vi "save_system_reference_meas_hdf.vi"(7 "Device Name":tag="DAQ2", 8 "HDF path":path, 9 "TxRxParams":T1={"sample rate"=1000000.0, "Transmit frequency"=25000.0, "Transmit amplitude"=1.577, "sample rate digital out"=40000.0, "TX cycles"=600, "sample rate DAQ1"=1000000.0, "Receive frequency"=75000.0, "Receive range"=1.0, "TX harmonics"=[50000.0, 75000.0, 100000.0, 125000.0, 150000.0, 175000.0, 200000.0, 225000.0]} {"TX harmonics" format="%#_6p"; "Receive frequency" format="%#_6p"; "sample rate DAQ1" format="%#_6p"; "sample rate digital out" format="%#_6p"; "Transmit frequency" format="%#_6p"; "sample rate" format="%#_6p"}, 11 "queue out 2":refnum<queue>) -> ()   [LabVIEW 2021]
uses:
  <vilib>/UPVI/lvhdf5/file.llb/LVH5F Operation.ctl
  <vilib>/Utility/miscctls.llb/LVRectTypeDef.ctl
  <vilib>/UPVI/lvhdf5/group.llb/H5G_obj_t.ctl
  <vilib>/UPVI/lvhdf5/dataset.llb/LVH5D Operation.ctl
  <vilib>/UPVI/lvhdf5/attribute.llb/Write Multiple Attributes.vi
  <vilib>/UPVI/lvhdf5/utility.llb/Select HDF5 Dialog.vi
  <vilib>/UPVI/lvhdf5/utility.llb/Select HDF5 Dialog (Object Only).vi
  <vilib>/UPVI/lvhdf5/dataset.llb/Simple H5Dwrite (Variant).vi
  <vilib>/UPVI/lvhdf5/attribute.llb/LVH5A Operation.ctl
  <vilib>/UPVI/lvhdf5/attribute.llb/LVH5 Write Attributes.xnode
  <vilib>/UPVI/lvhdf5/library.llb/HDF5 Ref.ctl
  <vilib>/UPVI/lvhdf5/dataset.llb/Simple H5Dwrite.xnode
  <resource>/objmgr/daqmx.rc
  <vilib>/UPVI/lvhdf5/attribute.llb/Cluster to Attribute Array.xnode
  <vilib>/UPVI/lvhdf5/identifier.llb/Not an HDF5 Refnum Constant.vi
  <vilib>/Utility/error.llb/Error Cluster From Error Code.vi
  <vilib>/UPVI/lvhdf5/dataset.llb/OpenCreateReplace Dataset by Element Type.vi
  <vilib>/UPVI/lvhdf5/dataspace.llb/H5Sselect_hyperslab.vi
  <vilib>/UPVI/lvhdf5/dataset.llb/H5Dwrite (Variant).vi
  <vilib>/UPVI/lvhdf5/dataset.llb/H5Dget_space.vi
  <vilib>/UPVI/lvhdf5/attribute.llb/private/LVH5AwriteWDTAttrs.vi
  <vilib>/UPVI/lvhdf5/dataspace.llb/H5Sclose.vi
  <vilib>/UPVI/lvhdf5/dataset.llb/H5Dclose.vi
  <vilib>/UPVI/lvhdf5/utility.llb/Select HDF5 Dialog (File and Object).vi
  <vilib>/UPVI/lvhdf5/library.llb/HDF5 Ref.lvclass
  <vilib>/Utility/Data Type/Get Type Information.vi
  <vilib>/Utility/Data Type/NI_Data Type.lvlib
  <vilib>/Utility/Data Type/Get Cluster Information.vi
panel:
  out "Run description":string
  out "index":i32
  out "f_harmonics":dbl[](array[numeric])
  out "x != 0?":bool
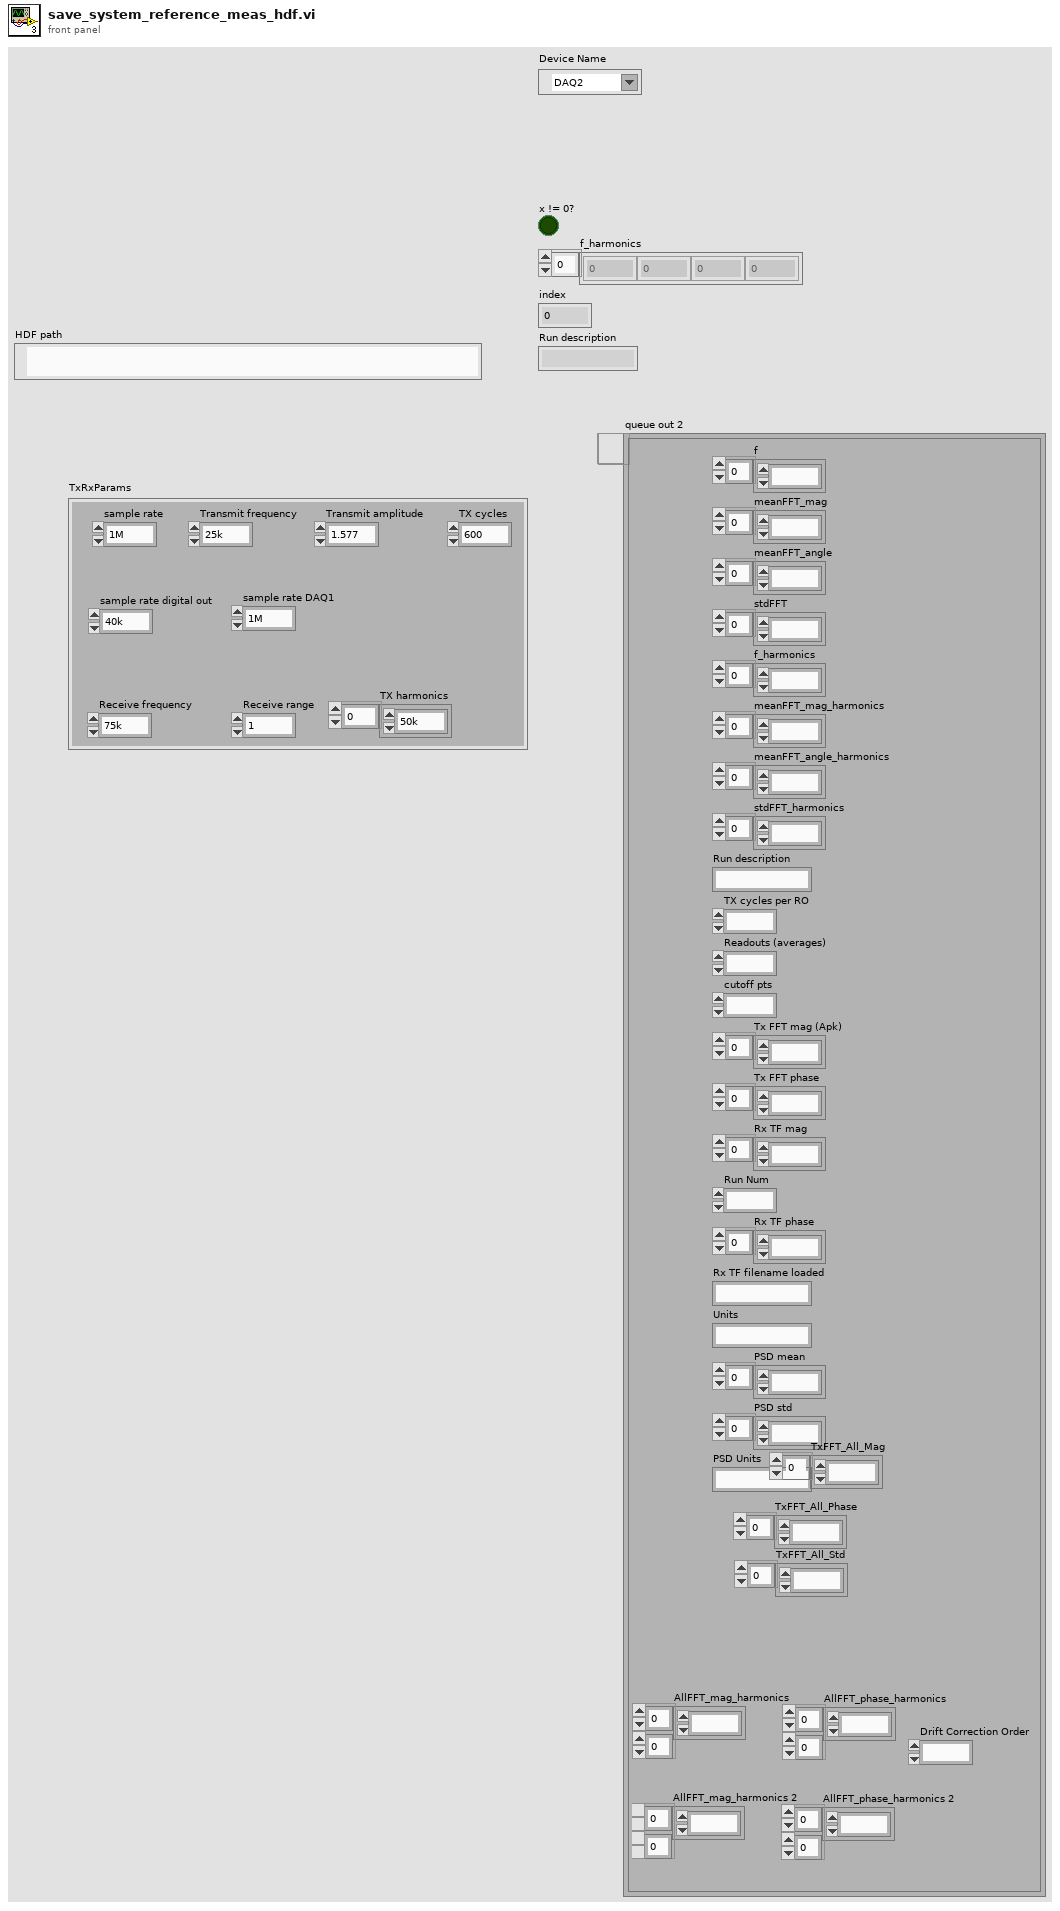
[diagram p1: front panel]
types:
  T1 = cluster{"sample rate":dbl, "Transmit frequency":dbl, "Transmit amplitude":dbl, "sample rate digital out":dbl, "TX cycles":i32, "sample rate DAQ1":dbl, "Receive frequency":dbl, "Receive range":dbl, "TX harmonics":dbl[]}
  T2 = typedef "LVH5F Operation.ctl" = enum16{"open", "open or create", "create or replace", "create or replace (with confirmation)", "create", "open (read only)"}
  T3 = typedef "LVRectTypeDef.ctl" = cluster{"Left":i16, "Top":i16, "Right":i16, "Bottom":i16}
  T4 = cluster{"Behavior":enum32{"Invalid", "Default", "Floating", "Floating/Auto-Hide", "Modal"}, "Position":T3, "Center":bool, "Title":string}
  T5 = typedef "LVH5D Operation.ctl" = enum16{"open", "replace", "create", "open or create", "create or replace", "create or replace with confirmation"}
  T6 = typedef "H5G_obj_t.ctl" = i32
  T7 = cluster{"Object Types (any)":T6[], "Object Pattern":string}
  T8 = cluster{"f":dbl[], "meanFFT_mag":dbl[], "meanFFT_angle":dbl[], "stdFFT":dbl[], "f_harmonics":dbl[], "meanFFT_mag_harmonics":dbl[], "meanFFT_angle_harmonics":dbl[], "stdFFT_harmonics":dbl[], "Run description":string, "TX cycles per RO":dbl, "Readouts (averages)":dbl, "cutoff pts":dbl, "Tx FFT mag (Apk)":dbl[], "Tx FFT phase":dbl[], "Rx TF mag":dbl[], "Run Num":i32, "Rx TF phase":dbl[], "Rx TF filename loaded":string, "Units":string, "PSD mean":dbl[], "PSD std":dbl[], "PSD Units":string, "TxFFT_All_Mag":dbl[], "TxFFT_All_Phase":dbl[], "TxFFT_All_Std":dbl[], "AllFFT_mag_harmonics":dbl[][], "AllFFT_phase_harmonics":dbl[][], "Drift Correction Order":dbl, "AllFFT_mag_harmonics 2":dbl[][], "AllFFT_phase_harmonics 2":dbl[][]}
  T9 = typedef "HDF5 Ref.ctl" = refnum<class "HDF5 Ref.lvclass">
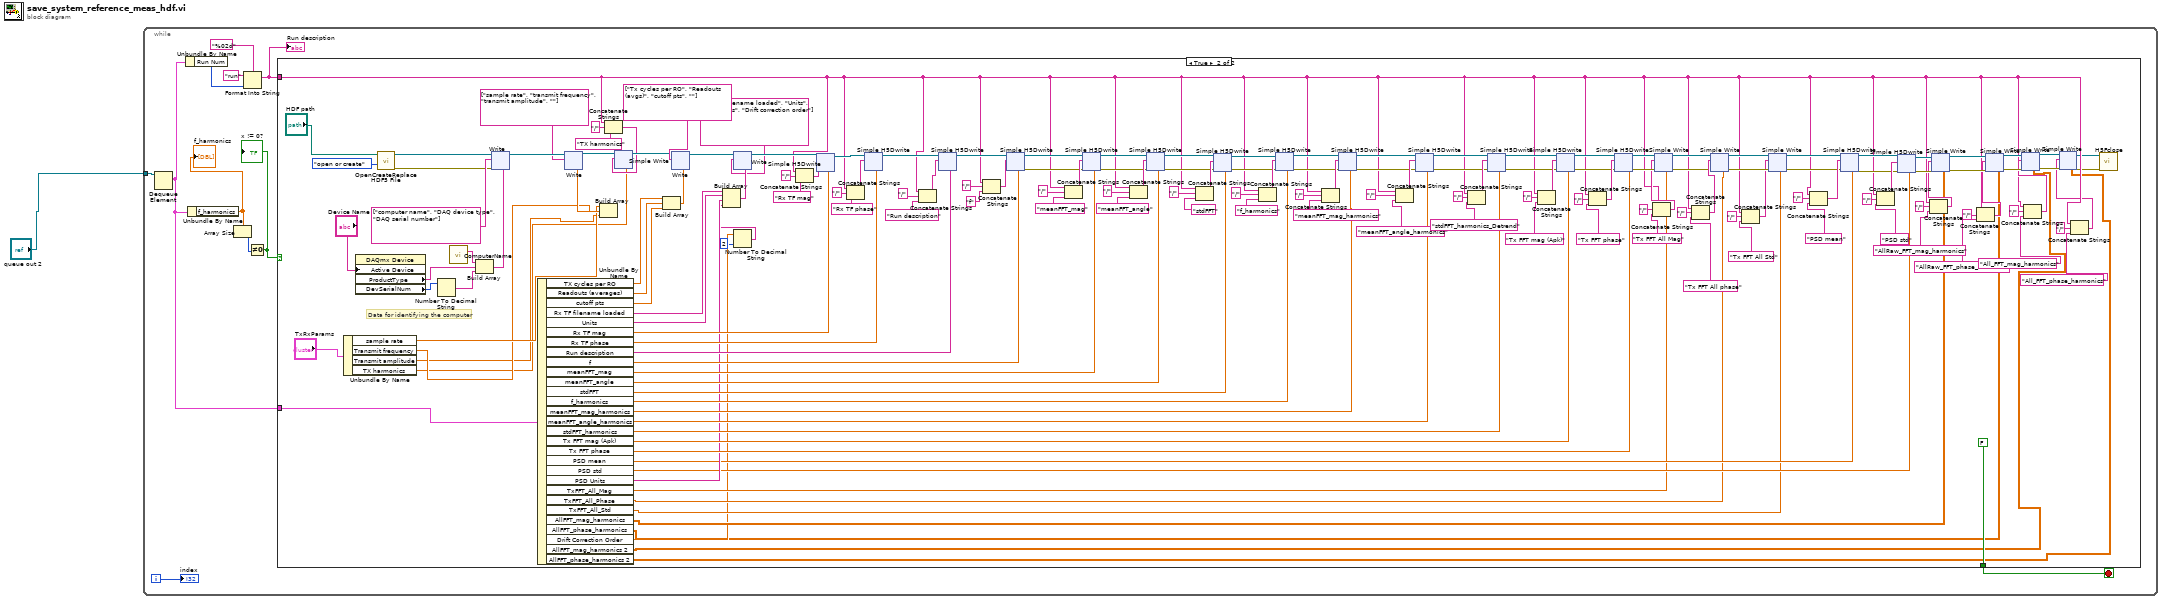
[diagram p0: block diagram]
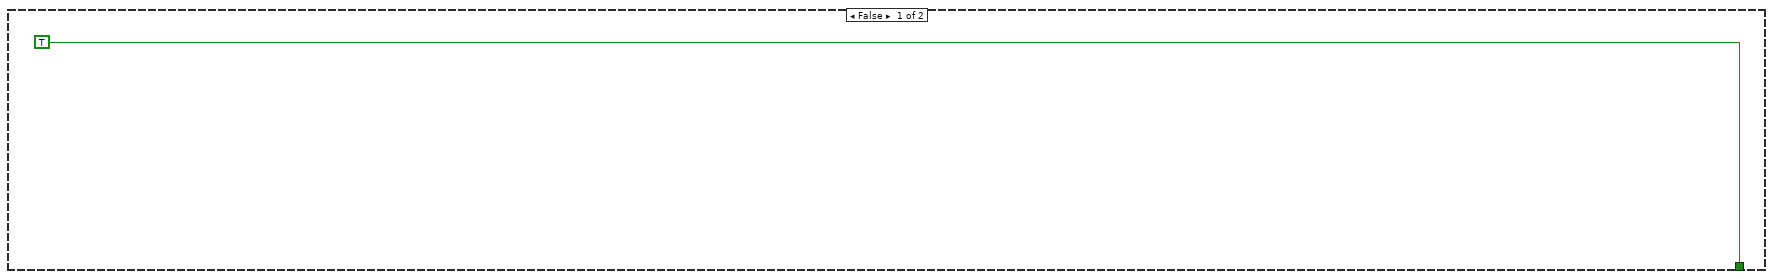
[diagram p2: hidden frame]
diagram:
  n1 = while {
    tunnel: "queue out 2" -> [w12]
    i -> [w8]
    stop <- w9 stop-if-true
    n2 = Dequeue Element(queue=w12) -> (element=w6:T8)  [unwired: 2 in, 3 out]
    n3 = Unbundle By Name(w6) -> ("Run Num"=w5:i32)
    n4 = Unbundle By Name(w6) -> ("f_harmonics"=w7:dbl[])
    "f_harmonics" <- w7
    n5 = Array Size(array=w7) -> (size(s)=w11:i32)
    n6 = Format Into String(format string="%02d", initial string="run", w5) -> (resulting string=w2:string)  [unwired: 1 in, 1 out]
    "Run description" <- w2
    n7 = Not Equal To 0?(x=w11) -> (x != 0?=w10:bool)
    "x != 0?" <- w10
    n8 = case shown="True" w10 {
      tunnel: w6 -> [_ w170]
      tunnel: [TRUE FALSE] -> w9
      tunnel: w2 -> [_ w19]
      frame False {
      }
      frame True {
        # "Data for identifying the computer"
        n9 = Unbundle By Name("TxRxParams") -> ("sample rate"=w70:dbl, "Transmit frequency"=w69:dbl, "Transmit amplitude"=w68:dbl, "TX harmonics"=w67:dbl[])
        n10 = property class="DAQmx Device"("Active Device"="Device Name") -> ("ProductType"=w181:string, "DevSerialNum"=w183:u32)  [unwired: 2 in, 2 out]
        n11 = call <vilib>:"OpenCreateReplace HDF5 File.vi"("function (open or create)"=LVH5F_Operation."open or create", "path"="HDF path") -> ("error out"=w175:errorcluster, "HDF5 Ref out"=w178:T9)  [unwired: 6 in]
        n12 = Number To Decimal String(number=w183) -> (decimal integer string=w182:string)  [unwired: 1 in]
        n13 = call "ComputerName.vi"() -> ("String/Binary data"=w180:string)  [unwired: 4 in, 1 out]
        n14 = Build Array(w180, w181, w182) -> (w177:string[])
        n15 = xnode "Write"("HDF5 Ref"=w178, "error in (no error)"=w175, "Name(s)"=string[] ["computer name", "DAQ device type", "DAQ serial number"], "Value(s)"=w177) -> ("HDF5 Ref out"=w126:T9)  [unwired: 1 in, 1 out]
        n16 = Unbundle By Name(w170) -> ("TX cycles per RO"=w112:dbl, "Readouts (averages)"=w111:dbl, "cutoff pts"=w110:dbl, "Rx TF filename loaded"=w88:string, "Units"=w90:string, "Rx TF mag"=w97:dbl[], "Rx TF phase"=w96:dbl[], "Run description"=w107:string, "f"=w140:dbl[], "meanFFT_mag"=w159:dbl[], "meanFFT_angle"=w158:dbl[], "stdFFT"=w157:dbl[], "f_harmonics"=w156:dbl[], "meanFFT_mag_harmonics"=w144:dbl[], "meanFFT_angle_harmonics"=w138:dbl[], "stdFFT_harmonics"=w137:dbl[], "Tx FFT mag (Apk)"=w120:dbl[], "Tx FFT phase"=w118:dbl[], "PSD mean"=w80:dbl[], "PSD std"=w79:dbl[], "PSD Units"=w81:string, "TxFFT_All_Mag"=w48:dbl[], "TxFFT_All_Phase"=w47:dbl[], "TxFFT_All_Std"=w46:dbl[], "AllFFT_mag_harmonics"=w33:dbl[][], "AllFFT_phase_harmonics"=w20:dbl[][], "Drift Correction Order"=w32:dbl, "AllFFT_mag_harmonics 2"=w15:dbl[][], "AllFFT_phase_harmonics 2"=w14:dbl[][])
        n17 = Build Array(w70, w69, w68) -> (w124:dbl[])
        n18 = xnode "Write"("HDF5 Ref"=w126, "Name(s)"=string[] ["sample rate", "transmit frequency", "transmit amplitude", ""], "Value(s)"=w124) -> ("HDF5 Ref out"=w86:T9)  [unwired: 2 in, 1 out]
        n19 = Concatenate Strings(w19, "/" ("string"), "TX harmonics" ("string")) -> (w82:string)
        n20 = xnode "Simple Write"("Dataset Path"=w82, "HDF5 Path or Ref"=w86, "Data"=w67) -> ("HDF5 Ref out"=w85:T9)  [unwired: 5 in, 2 out]
        n21 = Build Array(w112, w111, w110) -> (w109:dbl[])
        n22 = xnode "Write"("HDF5 Ref"=w85, "Name(s)"=string[] ["Tx cycles per RO", "Readouts (avgs)", "cutoff pts", ""], "Value(s)"=w109) -> ("HDF5 Ref out"=w92:T9)  [unwired: 2 in, 1 out]
        n23 = Number To Decimal String(number=w32, width (-)=i16 2) -> (decimal integer string=w30:string)
        n24 = Build Array(w88, w90, w81, w30) -> (w89:string[])
        n25 = xnode "Write"("HDF5 Ref"=w92, "Name(s)"=string[] ["Rx TF filename loaded", "Units", "PSD Units", "Drift correction order"], "Value(s)"=w89) -> ("HDF5 Ref out"=w91:T9)  [unwired: 2 in, 1 out]
        n26 = Concatenate Strings(w19, "/" ("string"), "Rx TF mag" ("string")) -> (w98:string)
        n27 = xnode "Simple H5Dwrite"("Dataset Path"=w98, "HDF5 Path or Ref"=w91, "Data"=w97) -> ("HDF5 Ref out"=w102:T9)  [unwired: 5 in, 2 out]
        n28 = Concatenate Strings(w19, "/" ("string"), "Rx TF phase" ("string")) -> (w93:string)
        n29 = xnode "Simple H5Dwrite"("Dataset Path"=w93, "HDF5 Path or Ref"=w102, "Data"=w96) -> ("HDF5 Ref out"=w101:T9)  [unwired: 5 in, 2 out]
        n30 = Concatenate Strings(w19, "/", "Run description" ("string")) -> (w103:string)
        n31 = xnode "Simple H5Dwrite"("Dataset Path"=w103, "HDF5 Path or Ref"=w101, "Data"=w107) -> ("HDF5 Ref out"=w106:T9)  [unwired: 5 in, 2 out]
        n32 = Concatenate Strings(w19, "/", "f" ("string")) -> (w141:string)
        n33 = xnode "Simple H5Dwrite"("Dataset Path"=w141, "HDF5 Path or Ref"=w106, "Data"=w140) -> ("HDF5 Ref out"=w113:T9, "error out"=w139:errorcluster)  [unwired: 5 in, 1 out]
        n34 = Concatenate Strings(w19, "/", "meanFFT_mag" ("string")) -> (w172:string)
        n35 = xnode "Simple H5Dwrite"("Dataset Path"=w172, "error in (no error)"=w139, "HDF5 Path or Ref"=w113, "Data"=w159) -> ("HDF5 Ref out"=w149:T9, "error out"=w148:errorcluster)  [unwired: 4 in, 1 out]
        n36 = Concatenate Strings(w19, "/", "meanFFT_angle" ("string")) -> (w168:string)
        n37 = xnode "Simple H5Dwrite"("Dataset Path"=w168, "error in (no error)"=w148, "HDF5 Path or Ref"=w149, "Data"=w158) -> ("HDF5 Ref out"=w150:T9, "error out"=w147:errorcluster)  [unwired: 4 in, 1 out]
        n38 = Concatenate Strings(w19, "/", "stdFFT" ("string")) -> (w164:string)
        n39 = xnode "Simple H5Dwrite"("Dataset Path"=w164, "error in (no error)"=w147, "HDF5 Path or Ref"=w150, "Data"=w157) -> ("HDF5 Ref out"=w151:T9, "error out"=w146:errorcluster)  [unwired: 4 in, 1 out]
        n40 = Concatenate Strings(w19, "/", "f_harmonics" ("string")) -> (w163:string)
        n41 = xnode "Simple H5Dwrite"("Dataset Path"=w163, "error in (no error)"=w146, "HDF5 Path or Ref"=w151, "Data"=w156) -> ("HDF5 Ref out"=w152:T9, "error out"=w145:errorcluster)  [unwired: 4 in, 1 out]
        n42 = Concatenate Strings(w19, "/", "meanFFT_mag_harmonics" ("string")) -> (w160:string)
        n43 = xnode "Simple H5Dwrite"("Dataset Path"=w160, "error in (no error)"=w145, "HDF5 Path or Ref"=w152, "Data"=w144) -> ("HDF5 Ref out"=w130:T9, "error out"=w128:errorcluster)  [unwired: 4 in, 1 out]
        n44 = Concatenate Strings(w19, "/", "meanFFT_angle_harmonics" ("string")) -> (w131:string)
        n45 = xnode "Simple H5Dwrite"("Dataset Path"=w131, "error in (no error)"=w128, "HDF5 Path or Ref"=w130, "Data"=w138) -> ("HDF5 Ref out"=w129:T9, "error out"=w127:errorcluster)  [unwired: 4 in, 1 out]
        n46 = Concatenate Strings(w19, "/", "stdFFT_harmonics_Detrend" ("string")) -> (w132:string)
        n47 = xnode "Simple H5Dwrite"("Dataset Path"=w132, "error in (no error)"=w127, "HDF5 Path or Ref"=w129, "Data"=w137) -> ("HDF5 Ref out"=w119:T9, "error out"=w51:errorcluster)  [unwired: 4 in, 1 out]
        n48 = Concatenate Strings(w19, "/", "Tx FFT mag (Apk)" ("string")) -> (w121:string)
        n49 = xnode "Simple H5Dwrite"("Dataset Path"=w121, "error in (no error)"=w51, "HDF5 Path or Ref"=w119, "Data"=w120) -> ("HDF5 Ref out"=w117:T9, "error out"=w50:errorcluster)  [unwired: 4 in, 1 out]
        n50 = Concatenate Strings(w19, "/" ("string"), "Tx FFT phase" ("string")) -> (w114:string)
        n51 = xnode "Simple H5Dwrite"("Dataset Path"=w114, "error in (no error)"=w50, "HDF5 Path or Ref"=w117, "Data"=w118) -> ("HDF5 Ref out"=w65:T9, "error out"=w66:errorcluster)  [unwired: 4 in, 1 out]
        n52 = Concatenate Strings(w19, "/" ("string"), "Tx FFT All Mag" ("string")) -> (w54:string)
        n53 = xnode "Simple Write"("Dataset Path"=w54, "error in (no error)"=w66, "HDF5 Path or Ref"=w65, "Data"=w48) -> ("HDF5 Ref out"=w63:T9, "error out"=w49:errorcluster)  [unwired: 4 in, 1 out]
        n54 = Concatenate Strings(w19, "/" ("string"), "Tx FFT All phase" ("string")) -> (w53:string)
        n55 = xnode "Simple Write"("Dataset Path"=w53, "error in (no error)"=w49, "HDF5 Path or Ref"=w63, "Data"=w47) -> ("HDF5 Ref out"=w62:T9, "error out"=w64:errorcluster)  [unwired: 4 in, 1 out]
        n56 = Concatenate Strings(w19, "/" ("string"), "Tx FFT All Std" ("string")) -> (w52:string)
        n57 = xnode "Simple Write"("Dataset Path"=w52, "error in (no error)"=w64, "HDF5 Path or Ref"=w62, "Data"=w46) -> ("HDF5 Ref out"=w61:T9, "error out"=w40:errorcluster)  [unwired: 4 in, 1 out]
        n58 = Concatenate Strings(w19, "/" ("string"), "PSD mean" ("string")) -> (w73:string)
        n59 = xnode "Simple H5Dwrite"("Dataset Path"=w73, "error in (no error)"=w40, "HDF5 Path or Ref"=w61, "Data"=w80) -> ("HDF5 Ref out"=w72:T9, "error out"=w41:errorcluster)  [unwired: 4 in, 1 out]
        n60 = Concatenate Strings(w19, "/" ("string"), "PSD std" ("string")) -> (w74:string)
        n61 = xnode "Simple H5Dwrite"("Dataset Path"=w74, "error in (no error)"=w41, "HDF5 Path or Ref"=w72, "Data"=w79) -> ("HDF5 Ref out"=w44:T9, "error out"=w45:errorcluster)  [unwired: 4 in, 1 out]
        n62 = Concatenate Strings(w19, "/" ("string"), "AllRaw_FFT_mag_harmonics" ("string")) -> (w35:string)
        n63 = xnode "Simple Write"("Dataset Path"=w35, "error in (no error)"=w45, "HDF5 Path or Ref"=w44, "Data"=w33) -> ("HDF5 Ref out"=w42:T9, "error out"=w43:errorcluster)  [unwired: 4 in, 1 out]
        n64 = Concatenate Strings(w19, "/" ("string"), "AllRaw_FFT_phase_harmonics" ("string")) -> (w34:string)
        n65 = xnode "Simple Write"("Dataset Path"=w34, "error in (no error)"=w43, "HDF5 Path or Ref"=w42, "Data"=w20) -> ("HDF5 Ref out"=w28:T9, "error out"=w27:errorcluster)  [unwired: 4 in, 1 out]
        n66 = Concatenate Strings(w19, "/" ("string"), "All_FFT_mag_harmonics" ("string")) -> (w25:string)
        n67 = xnode "Simple Write"("Dataset Path"=w25, "error in (no error)"=w27, "HDF5 Path or Ref"=w28, "Data"=w15) -> ("HDF5 Ref out"=w24:T9, "error out"=w23:errorcluster)  [unwired: 4 in, 1 out]
        n68 = Concatenate Strings(w19, "/" ("string"), "All_FFT_phase_harmonics" ("string")) -> (w16:string)
        n69 = xnode "Simple Write"("Dataset Path"=w16, "error in (no error)"=w23, "HDF5 Path or Ref"=w24, "Data"=w14) -> ("HDF5 Ref out"=w18:T9, "error out"=w17:errorcluster)  [unwired: 4 in, 1 out]
        n70 = call <vilib>:"H5Fclose.vi"("error in (no error)"=w17, "HDF5 Ref"=w18) -> ()  [unwired: 7 in, 1 out]
      }
    }
    "index" <- w8
  }
